vi "Dresden Edit Recipe(in).vi"() -> ()   [LabVIEW 2009] (continued)
                n2220 = local write "R Cmb Ch3 Target material"("Zn" ("R DC Target material")) -> ()
              }
              frame #97 {
                n2221 = local write "R Cmb Ch3 Target material"("ZnO" ("R DC Target material")) -> ()
              }
              frame #98 {
                n2222 = local write "R Cmb Ch3 Target material"("ZnSe" ("R DC Target material")) -> ()
              }
              frame #99 {
                n2223 = local write "R Cmb Ch3 Target material"("ZnS" ("R DC Target material")) -> ()
              }
              frame #100 {
                n2224 = local write "R Cmb Ch3 Target material"("Zr" ("R DC Target material")) -> ()
              }
              frame #101 {
                n2225 = local write "R Cmb Ch3 Target material"("ZrO2" ("R DC Target material")) -> ()
              }
              frame #102 {
                n2226 = local write "R Cmb Ch3 Target material"("Si3N4" ("R DC Target material")) -> ()
              }
              frame #103 {
                n2227 = local write "R Cmb Ch3 Target material"("ITO" ("R DC Target material")) -> ()
              }
              frame #104 {
                n2228 = local write "R Cmb Ch3 Target material"("PbI2" ("R DC Target material")) -> ()
              }
            }
            n2229 = local read "R Cmb Step9 Coating Power Active"() -> (w824:bool)
            n2230 = local read "R Cmb Step8 Coating Power Active"() -> (w825:bool)
            n2231 = case shown="True" w827 {
              frame #0 {
                w1044 = FALSE ("R Cmb Step3 Coating Power Active")
                n2232 = local write "R Cmb Step7 Coating Power Active"(w1044) -> ()
                n2233 = local write "R Cmb Step8 Coating Power Active"(w1044) -> ()
                n2234 = local write "R Cmb Step9 Coating Power Active"(w1044) -> ()
                n2235 = local write "R Cmb Step10 Coating Power Active"(w1044) -> ()
              }
              frame #1 {
                n2236 = local read "R Cmb Step7 Coating Power Active"() -> (w1045:bool)
                n2237 = case shown="False" w1045 {
                  frame #0 {
                    w1046 = 0.0 ("R Cmb Ch2 Step7 Coating Power")
                    w1047 = T5."Disabled and Grayed Out" ("Disabled")
                    n2238 = local write "R Cmb Ch3 Step7 Coating Power"(w1046) -> ()
                    n2239 = local write "R Cmb Ch2 Step7 Coating Power"(w1046) -> ()
                    n2240 = local write "R Cmb Interval length 7"(w1046) -> ()
                    n2241 = property on="R Cmb Ch3 Step7 Coating Power" class="DigNum (strict)"("DisabledEnum"=w1047) -> ()  [unwired: 2 in, 2 out]
                    n2242 = property on="R Cmb Interval length 7" class="DigNum (strict)"("DisabledEnum"=w1047) -> ()  [unwired: 2 in, 2 out]
                    n2243 = property on="R Cmb Ch2 Step7 Coating Power" class="DigNum (strict)"("DisabledEnum"=w1047) -> ()  [unwired: 2 in, 2 out]
                  }
                  frame #1 {
                    w1048 = T5."Enabled" ("Disabled")
                    n2244 = property on="R Cmb Ch3 Step7 Coating Power" class="DigNum (strict)"("DisabledEnum"=w1048) -> ()  [unwired: 2 in, 2 out]
                    n2245 = property on="R Cmb Interval length 7" class="DigNum (strict)"("DisabledEnum"=w1048) -> ()  [unwired: 2 in, 2 out]
                    n2246 = property on="R Cmb Ch2 Step7 Coating Power" class="DigNum (strict)"("DisabledEnum"=w1048) -> ()  [unwired: 2 in, 2 out]
                  }
                }
              }
            }
            n2247 = case shown="True" w826 {
              frame #0 {
                w1039 = FALSE ("R Cmb Step3 Coating Power Active")
                n2248 = local write "R Cmb Step8 Coating Power Active"(w1039) -> ()
                n2249 = local write "R Cmb Step9 Coating Power Active"(w1039) -> ()
                n2250 = local write "R Cmb Step10 Coating Power Active"(w1039) -> ()
              }
              frame #1 {
                n2251 = local read "R Cmb Step8 Coating Power Active"() -> (w1040:bool)
                n2252 = case shown="False" w1040 {
                  frame #0 {
                    w1041 = 0.0 ("R Cmb Ch2 Step8 Coating Power")
                    w1042 = T5."Disabled and Grayed Out" ("Disabled")
                    n2253 = local write "R Cmb Ch3 Step8 Coating Power"(w1041) -> ()
                    n2254 = local write "R Cmb Ch2 Step8 Coating Power"(w1041) -> ()
                    n2255 = local write "R Cmb Interval length 8"(w1041) -> ()
                    n2256 = property on="R Cmb Ch2 Step8 Coating Power" class="DigNum (strict)"("DisabledEnum"=w1042) -> ()  [unwired: 2 in, 2 out]
                    n2257 = property on="R Cmb Ch3 Step8 Coating Power" class="DigNum (strict)"("DisabledEnum"=w1042) -> ()  [unwired: 2 in, 2 out]
                    n2258 = property on="R Cmb Interval length 8" class="DigNum (strict)"("DisabledEnum"=w1042) -> ()  [unwired: 2 in, 2 out]
                  }
                  frame #1 {
                    w1043 = T5."Enabled" ("Disabled")
                    n2259 = property on="R Cmb Ch2 Step8 Coating Power" class="DigNum (strict)"("DisabledEnum"=w1043) -> ()  [unwired: 2 in, 2 out]
                    n2260 = property on="R Cmb Ch3 Step8 Coating Power" class="DigNum (strict)"("DisabledEnum"=w1043) -> ()  [unwired: 2 in, 2 out]
                    n2261 = property on="R Cmb Interval length 8" class="DigNum (strict)"("DisabledEnum"=w1043) -> ()  [unwired: 2 in, 2 out]
                  }
                }
              }
            }
            n2262 = case shown="True" w828 {
              frame #0 {
                w1049 = FALSE ("R Cmb Step3 Coating Power Active")
                n2263 = local write "R Cmb Step6 Coating Power Active"(w1049) -> ()
                n2264 = local write "R Cmb Step7 Coating Power Active"(w1049) -> ()
                n2265 = local write "R Cmb Step8 Coating Power Active"(w1049) -> ()
                n2266 = local write "R Cmb Step9 Coating Power Active"(w1049) -> ()
                n2267 = local write "R Cmb Step10 Coating Power Active"(w1049) -> ()
              }
              frame #1 {
                n2268 = local read "R Cmb Step6 Coating Power Active"() -> (w1050:bool)
                n2269 = case shown="False" w1050 {
                  frame #0 {
                    w1051 = 0.0 ("R Cmb Ch2 Step6 Coating Power")
                    w1052 = T5."Disabled and Grayed Out" ("Disabled")
                    n2270 = local write "R Cmb Ch2 Step6 Coating Power"(w1051) -> ()
                    n2271 = local write "R Cmb Ch3 Step6 Coating Power"(w1051) -> ()
                    n2272 = local write "R Cmb Interval length 6"(w1051) -> ()
                    n2273 = property on="R Cmb Ch2 Step6 Coating Power" class="DigNum (strict)"("DisabledEnum"=w1052) -> ()  [unwired: 2 in, 2 out]
                    n2274 = property on="R Cmb Ch3 Step6 Coating Power" class="DigNum (strict)"("DisabledEnum"=w1052) -> ()  [unwired: 2 in, 2 out]
                    n2275 = property on="R Cmb Interval length 6" class="DigNum (strict)"("DisabledEnum"=w1052) -> ()  [unwired: 2 in, 2 out]
                  }
                  frame #1 {
                    w1053 = T5."Enabled" ("Disabled")
                    n2276 = property on="R Cmb Ch2 Step6 Coating Power" class="DigNum (strict)"("DisabledEnum"=w1053) -> ()  [unwired: 2 in, 2 out]
                    n2277 = property on="R Cmb Ch3 Step6 Coating Power" class="DigNum (strict)"("DisabledEnum"=w1053) -> ()  [unwired: 2 in, 2 out]
                    n2278 = property on="R Cmb Interval length 6" class="DigNum (strict)"("DisabledEnum"=w1053) -> ()  [unwired: 2 in, 2 out]
                  }
                }
              }
            }
            n2279 = case shown="True" w824 {
              frame #0 {
                n2280 = local write "R Cmb Step10 Coating Power Active"(FALSE ("R Cmb Step3 Coating Power Active")) -> ()
              }
              frame #1 {
                n2281 = local read "R Cmb Step10 Coating Power Active"() -> (w1035:bool)
                n2282 = case shown="False" w1035 {
                  frame #0 {
                    w1036 = 0.0 ("R Cmb Ch2 Step10 Coating Power")
                    w1037 = T5."Disabled and Grayed Out" ("Disabled")
                    n2283 = local write "R Cmb Ch2 Step10 Coating Power"(w1036) -> ()
                    n2284 = local write "R Cmb Ch3 Step10 Coating Power"(w1036) -> ()
                    n2285 = local write "R Cmb Interval length 10"(w1036) -> ()
                    n2286 = property on="R Cmb Ch2 Step10 Coating Power" class="DigNum (strict)"("DisabledEnum"=w1037) -> ()  [unwired: 2 in, 2 out]
                    n2287 = property on="R Cmb Ch3 Step10 Coating Power" class="DigNum (strict)"("DisabledEnum"=w1037) -> ()  [unwired: 2 in, 2 out]
                    n2288 = property on="R Cmb Interval length 10" class="DigNum (strict)"("DisabledEnum"=w1037) -> ()  [unwired: 2 in, 2 out]
                  }
                  frame #1 {
                    w1038 = T5."Enabled" ("Disabled")
                    n2289 = property on="R Cmb Ch2 Step10 Coating Power" class="DigNum (strict)"("DisabledEnum"=w1038) -> ()  [unwired: 2 in, 2 out]
                    n2290 = property on="R Cmb Ch3 Step10 Coating Power" class="DigNum (strict)"("DisabledEnum"=w1038) -> ()  [unwired: 2 in, 2 out]
                    n2291 = property on="R Cmb Interval length 10" class="DigNum (strict)"("DisabledEnum"=w1038) -> ()  [unwired: 2 in, 2 out]
                  }
                }
              }
            }
            n2292 = case shown="True" w825 {
              frame #0 {
                w1029 = FALSE ("R Cmb Step3 Coating Power Active")
                n2293 = local write "R Cmb Step9 Coating Power Active"(w1029) -> ()
                n2294 = local write "R Cmb Step10 Coating Power Active"(w1029) -> ()
              }
              frame #1 {
                n2295 = local read "R Cmb Step9 Coating Power Active"() -> (w1030:bool)
                n2296 = case shown="False" w1030 {
                  frame #0 {
                    w1031 = 0.0 ("R Cmb Ch2 Step9 Coating Power")
                    w1032 = T5."Disabled and Grayed Out" ("Disabled")
                    n2297 = local write "R Cmb Ch3 Step9 Coating Power"(w1031) -> ()
                    n2298 = local write "R Cmb Ch2 Step9 Coating Power"(w1031) -> ()
                    n2299 = local write "R Cmb Interval length 9"(w1031) -> ()
                    n2300 = property on="R Cmb Ch2 Step9 Coating Power" class="DigNum (strict)"("DisabledEnum"=w1032) -> ()  [unwired: 2 in, 2 out]
                    n2301 = property on="R Cmb Ch3 Step9 Coating Power" class="DigNum (strict)"("DisabledEnum"=w1032) -> ()  [unwired: 2 in, 2 out]
                    n2302 = property on="R Cmb Interval length 9" class="DigNum (strict)"("DisabledEnum"=w1032) -> ()  [unwired: 2 in, 2 out]
                  }
                  frame #1 {
                    w1033 = T5."Enabled" ("Disabled")
                    n2303 = property on="R Cmb Ch2 Step9 Coating Power" class="DigNum (strict)"("DisabledEnum"=w1033) -> ()  [unwired: 2 in, 2 out]
                    n2304 = property on="R Cmb Ch3 Step9 Coating Power" class="DigNum (strict)"("DisabledEnum"=w1033) -> ()  [unwired: 2 in, 2 out]
                    n2305 = property on="R Cmb Interval length 9" class="DigNum (strict)"("DisabledEnum"=w1033) -> ()  [unwired: 2 in, 2 out]
                  }
                }
              }
            }
            n2306 = Or(x=w853, y="Cancel") -> (x .or. y?=w851:bool)
          }
        }
        frame #1 {
        }
      }
    }
  }
  "OKTO" <- w1
  n2307 = invoke class="VI" method="Default Vals.Reinit All"() -> (error out=w4:errorcluster)  [unwired: 3 in, 2 out]
  n2308 = property on="Recipe Name" class="Str"(error in=w4, "Key Focus"=TRUE) -> ()  [unwired: 1 in, 2 out]
  n2309 = case shown="True" w1 {
    tunnel: [errorcluster {"status"=FALSE, "code"=0, "source"=""} ("error out") w2514] -> w2
    frame #0 {
    }
    frame #1 {
      n2310 = stacked-sequence {
        seq-local: [w2521 _] -> [_ w2718]
        seq-local: [w2520 _] -> [_ w2714]
        seq-local: [w2519 _] -> [_ w2720]
        seq-local: [w2518 _] -> [_ w2715]
        seq-local: [w2516 _] -> [_ w2708]
        seq-local: [w2515 _] -> [_ w2711]
        tunnel: [_ w2719] -> w2514
        tunnel: [_ w2713] -> _
        tunnel: [_ w2710] -> _
        frame #0 {
          n2311 = File Dialog(9:"Recipe Name", 11:path "D:/System Files/Recipe" ("start path")) -> (3:w2528:path)  [unwired: 2 in, 6 out]
          n2312 = Build Path(base path=path "D:/System Files/Recipe" ("start path"), name or relative path="Recipe Name") -> (appended path=w2527:path)
          n2313 = Open/Create/Replace File(file path (use dialog)=w2527, operation (0:open)=T6."replace or create", access (0:read/write)=enum16{"read/write", "read-only", "write-only"}."read/write") -> (refnum out=w2518:refnum<file>, cancelled=w2525:bool, error out=w2523:errorcluster)  [unwired: 3 in]
          n2314 = Open/Create/Replace File(file path (use dialog)=w2528, operation (0:open)=T6."replace or create", access (0:read/write)=enum16{"read/write", "read-only", "write-only"}."read/write") -> (refnum out=w2519:refnum<file>, cancelled=w2531:bool, error out=w2533:errorcluster)  [unwired: 3 in]
          n2315 = stacked-sequence {
            tunnel: "Recipe Name" -> [_ w2539 _]
            tunnel: [_ w2538 _] -> w2516
            tunnel: [_ w2537 _] -> w2515
            frame #0 {
              n2316 = Wait (ms)(milliseconds to wait=u32 50) -> ()  [unwired: 1 out]
              n2317 = dll-call lib="kernel32.dll" fn="SetFileAttributesA"("lpFileName"="D:\\System Files\\Recipe Archive", "dwFileAttributes"=u32 128) -> ()  [unwired: 6 in, 2 out]
            }
            frame #1 {
              n2318 = Build Path(base path=path "D:/System Files/Recipe Archive" ("start path"), name or relative path=w2539) -> (appended path=w2540:path)
              n2319 = Open/Create/Replace File(file path (use dialog)=w2540, operation (0:open)=T6."replace or create", access (0:read/write)=enum16{"read/write", "read-only", "write-only"}."read/write") -> (refnum out=w2538:refnum<file>, cancelled=w2542:bool, error out=w2544:errorcluster)  [unwired: 3 in]
              n2320 = case shown="True" w2542 {
                tunnel: w2538 -> [_ w2549]
                tunnel: w2544 -> [_ w2548]
                tunnel: [errorcluster {"status"=FALSE, "code"=0, "source"=""} ("error out") w2547] -> w2537
                frame #0 {
                }
                frame #1 {
                  n2321 = Close File(refnum=w2549, error in=w2548) -> (error out=w2547:errorcluster)  [unwired: 1 out]
                }
              }
            }
            frame #2 {
              n2322 = Wait (ms)(milliseconds to wait=u32 50) -> ()  [unwired: 1 out]
              n2323 = dll-call lib="kernel32.dll" fn="SetFileAttributesA"("lpFileName"="D:\\System Files\\Recipe Archive", "dwFileAttributes"=u32 2) -> ()  [unwired: 6 in, 2 out]
            }
          }
          n2324 = case shown="False" w2525 {
            tunnel: w2518 -> [_ w2556]
            tunnel: w2523 -> [_ w2555]
            tunnel: [errorcluster {"status"=FALSE, "code"=0, "source"=""} ("error out") w2554] -> w2520
            frame #0 {
            }
            frame #1 {
              n2325 = Close File(refnum=w2556, error in=w2555) -> (error out=w2554:errorcluster)  [unwired: 1 out]
            }
          }
          n2326 = case shown="True" w2531 {
            tunnel: w2519 -> [_ w2560]
            tunnel: w2533 -> [_ w2559]
            tunnel: [errorcluster {"status"=FALSE, "code"=0, "source"=""} ("error out") w2558] -> w2521
            frame #0 {
            }
            frame #1 {
              n2327 = Close File(refnum=w2560, error in=w2559) -> (error out=w2558:errorcluster)  [unwired: 1 out]
            }
          }
        }
        frame #1 {
          n2328 = stacked-sequence {
            tunnel: [w2723 _ _ _ _ _ _ _ _ _ _ _ _ _ _ _ _ _ _ _ _ _ _ _ _ _ _ _ _ _ _ _ _ _ _ _ _ _ _ _ _ _ _ _ _ _ _ _ _ _ _ _ _ _ _ _ _ _ _ _ _ _ _ _ _ _ _ _ _ _ _ _ _ _ _ _ _ _ _ _ _ _ _ _ _ _ _ _ _ _ _ _ _ _ _ _ _ _ _ _ _ _ _ _ _ _ _ _ _ _ _ _ _ _ _ _ _ _ _ _ _ _ _ _ _ _ _ _ _ _ _ _ _ _ _ _ _ _ _ _ _ _ _ _ _ _] -> w2706
            tunnel: [_ w2730 _ _ _ _ _ _ _ _ _ _ _ _ _ _ _ _ _ _ _ _ _ _ _ _ _ _ _ _ _ _ _ _ _ _ _ _ _ _ _ _ _ _ _ _ _ _ _ _ _ _ _ _ _ _ _ _ _ _ _ _ _ _ _ _ _ _ _ _ _ _ _ _ _ _ _ _ _ _ _ _ _ _ _ _ _ _ _ _ _ _ _ _ _ _ _ _ _ _ _ _ _ _ _ _ _ _ _ _ _ _ _ _ _ _ _ _ _ _ _ _ _ _ _ _ _ _ _ _ _ _ _ _ _ _ _ _ _ _ _ _ _ _ _ _] -> w2705
            tunnel: [_ _ w2737 _ _ _ _ _ _ _ _ _ _ _ _ _ _ _ _ _ _ _ _ _ _ _ _ _ _ _ _ _ _ _ _ _ _ _ _ _ _ _ _ _ _ _ _ _ _ _ _ _ _ _ _ _ _ _ _ _ _ _ _ _ _ _ _ _ _ _ _ _ _ _ _ _ _ _ _ _ _ _ _ _ _ _ _ _ _ _ _ _ _ _ _ _ _ _ _ _ _ _ _ _ _ _ _ _ _ _ _ _ _ _ _ _ _ _ _ _ _ _ _ _ _ _ _ _ _ _ _ _ _ _ _ _ _ _ _ _ _ _ _ _ _ _] -> w2704
            tunnel: [_ _ _ w2746 _ _ _ _ _ _ _ _ _ _ _ _ _ _ _ _ _ _ _ _ _ _ _ _ _ _ _ _ _ _ _ _ _ _ _ _ _ _ _ _ _ _ _ _ _ _ _ _ _ _ _ _ _ _ _ _ _ _ _ _ _ _ _ _ _ _ _ _ _ _ _ _ _ _ _ _ _ _ _ _ _ _ _ _ _ _ _ _ _ _ _ _ _ _ _ _ _ _ _ _ _ _ _ _ _ _ _ _ _ _ _ _ _ _ _ _ _ _ _ _ _ _ _ _ _ _ _ _ _ _ _ _ _ _ _ _ _ _ _ _ _ _] -> w2703
            tunnel: [_ _ _ _ w2755 _ _ _ _ _ _ _ _ _ _ _ _ _ _ _ _ _ _ _ _ _ _ _ _ _ _ _ _ _ _ _ _ _ _ _ _ _ _ _ _ _ _ _ _ _ _ _ _ _ _ _ _ _ _ _ _ _ _ _ _ _ _ _ _ _ _ _ _ _ _ _ _ _ _ _ _ _ _ _ _ _ _ _ _ _ _ _ _ _ _ _ _ _ _ _ _ _ _ _ _ _ _ _ _ _ _ _ _ _ _ _ _ _ _ _ _ _ _ _ _ _ _ _ _ _ _ _ _ _ _ _ _ _ _ _ _ _ _ _ _ _] -> w2702
            tunnel: [_ _ _ _ _ w2759 _ _ _ _ _ _ _ _ _ _ _ _ _ _ _ _ _ _ _ _ _ _ _ _ _ _ _ _ _ _ _ _ _ _ _ _ _ _ _ _ _ _ _ _ _ _ _ _ _ _ _ _ _ _ _ _ _ _ _ _ _ _ _ _ _ _ _ _ _ _ _ _ _ _ _ _ _ _ _ _ _ _ _ _ _ _ _ _ _ _ _ _ _ _ _ _ _ _ _ _ _ _ _ _ _ _ _ _ _ _ _ _ _ _ _ _ _ _ _ _ _ _ _ _ _ _ _ _ _ _ _ _ _ _ _ _ _ _ _ _] -> w2701
            tunnel: [_ _ _ _ _ _ w2765 _ _ _ _ _ _ _ _ _ _ _ _ _ _ _ _ _ _ _ _ _ _ _ _ _ _ _ _ _ _ _ _ _ _ _ _ _ _ _ _ _ _ _ _ _ _ _ _ _ _ _ _ _ _ _ _ _ _ _ _ _ _ _ _ _ _ _ _ _ _ _ _ _ _ _ _ _ _ _ _ _ _ _ _ _ _ _ _ _ _ _ _ _ _ _ _ _ _ _ _ _ _ _ _ _ _ _ _ _ _ _ _ _ _ _ _ _ _ _ _ _ _ _ _ _ _ _ _ _ _ _ _ _ _ _ _ _ _ _] -> w2700
            tunnel: [_ _ _ _ _ _ _ w2771 _ _ _ _ _ _ _ _ _ _ _ _ _ _ _ _ _ _ _ _ _ _ _ _ _ _ _ _ _ _ _ _ _ _ _ _ _ _ _ _ _ _ _ _ _ _ _ _ _ _ _ _ _ _ _ _ _ _ _ _ _ _ _ _ _ _ _ _ _ _ _ _ _ _ _ _ _ _ _ _ _ _ _ _ _ _ _ _ _ _ _ _ _ _ _ _ _ _ _ _ _ _ _ _ _ _ _ _ _ _ _ _ _ _ _ _ _ _ _ _ _ _ _ _ _ _ _ _ _ _ _ _ _ _ _ _ _ _] -> w2699
            tunnel: [_ _ _ _ _ _ _ _ w2777 _ _ _ _ _ _ _ _ _ _ _ _ _ _ _ _ _ _ _ _ _ _ _ _ _ _ _ _ _ _ _ _ _ _ _ _ _ _ _ _ _ _ _ _ _ _ _ _ _ _ _ _ _ _ _ _ _ _ _ _ _ _ _ _ _ _ _ _ _ _ _ _ _ _ _ _ _ _ _ _ _ _ _ _ _ _ _ _ _ _ _ _ _ _ _ _ _ _ _ _ _ _ _ _ _ _ _ _ _ _ _ _ _ _ _ _ _ _ _ _ _ _ _ _ _ _ _ _ _ _ _ _ _ _ _ _ _] -> w2698
            tunnel: [_ _ _ _ _ _ _ _ _ w2783 _ _ _ _ _ _ _ _ _ _ _ _ _ _ _ _ _ _ _ _ _ _ _ _ _ _ _ _ _ _ _ _ _ _ _ _ _ _ _ _ _ _ _ _ _ _ _ _ _ _ _ _ _ _ _ _ _ _ _ _ _ _ _ _ _ _ _ _ _ _ _ _ _ _ _ _ _ _ _ _ _ _ _ _ _ _ _ _ _ _ _ _ _ _ _ _ _ _ _ _ _ _ _ _ _ _ _ _ _ _ _ _ _ _ _ _ _ _ _ _ _ _ _ _ _ _ _ _ _ _ _ _ _ _ _ _] -> w2697
            tunnel: [_ _ _ _ _ _ _ _ _ _ w2789 _ _ _ _ _ _ _ _ _ _ _ _ _ _ _ _ _ _ _ _ _ _ _ _ _ _ _ _ _ _ _ _ _ _ _ _ _ _ _ _ _ _ _ _ _ _ _ _ _ _ _ _ _ _ _ _ _ _ _ _ _ _ _ _ _ _ _ _ _ _ _ _ _ _ _ _ _ _ _ _ _ _ _ _ _ _ _ _ _ _ _ _ _ _ _ _ _ _ _ _ _ _ _ _ _ _ _ _ _ _ _ _ _ _ _ _ _ _ _ _ _ _ _ _ _ _ _ _ _ _ _ _ _ _ _] -> w2696
            tunnel: [_ _ _ _ _ _ _ _ _ _ _ w2796 _ _ _ _ _ _ _ _ _ _ _ _ _ _ _ _ _ _ _ _ _ _ _ _ _ _ _ _ _ _ _ _ _ _ _ _ _ _ _ _ _ _ _ _ _ _ _ _ _ _ _ _ _ _ _ _ _ _ _ _ _ _ _ _ _ _ _ _ _ _ _ _ _ _ _ _ _ _ _ _ _ _ _ _ _ _ _ _ _ _ _ _ _ _ _ _ _ _ _ _ _ _ _ _ _ _ _ _ _ _ _ _ _ _ _ _ _ _ _ _ _ _ _ _ _ _ _ _ _ _ _ _ _ _] -> w2695
            tunnel: [_ _ _ _ _ _ _ _ _ _ _ _ w2801 _ _ _ _ _ _ _ _ _ _ _ _ _ _ _ _ _ _ _ _ _ _ _ _ _ _ _ _ _ _ _ _ _ _ _ _ _ _ _ _ _ _ _ _ _ _ _ _ _ _ _ _ _ _ _ _ _ _ _ _ _ _ _ _ _ _ _ _ _ _ _ _ _ _ _ _ _ _ _ _ _ _ _ _ _ _ _ _ _ _ _ _ _ _ _ _ _ _ _ _ _ _ _ _ _ _ _ _ _ _ _ _ _ _ _ _ _ _ _ _ _ _ _ _ _ _ _ _ _ _ _ _ _] -> w2694
            tunnel: [_ _ _ _ _ _ _ _ _ _ _ _ _ w2809 _ _ _ _ _ _ _ _ _ _ _ _ _ _ _ _ _ _ _ _ _ _ _ _ _ _ _ _ _ _ _ _ _ _ _ _ _ _ _ _ _ _ _ _ _ _ _ _ _ _ _ _ _ _ _ _ _ _ _ _ _ _ _ _ _ _ _ _ _ _ _ _ _ _ _ _ _ _ _ _ _ _ _ _ _ _ _ _ _ _ _ _ _ _ _ _ _ _ _ _ _ _ _ _ _ _ _ _ _ _ _ _ _ _ _ _ _ _ _ _ _ _ _ _ _ _ _ _ _ _ _ _] -> w2693
            tunnel: [_ _ _ _ _ _ _ _ _ _ _ _ _ _ w2815 _ _ _ _ _ _ _ _ _ _ _ _ _ _ _ _ _ _ _ _ _ _ _ _ _ _ _ _ _ _ _ _ _ _ _ _ _ _ _ _ _ _ _ _ _ _ _ _ _ _ _ _ _ _ _ _ _ _ _ _ _ _ _ _ _ _ _ _ _ _ _ _ _ _ _ _ _ _ _ _ _ _ _ _ _ _ _ _ _ _ _ _ _ _ _ _ _ _ _ _ _ _ _ _ _ _ _ _ _ _ _ _ _ _ _ _ _ _ _ _ _ _ _ _ _ _ _ _ _ _ _] -> w2692
            tunnel: [_ _ _ _ _ _ _ _ _ _ _ _ _ _ _ w2822 _ _ _ _ _ _ _ _ _ _ _ _ _ _ _ _ _ _ _ _ _ _ _ _ _ _ _ _ _ _ _ _ _ _ _ _ _ _ _ _ _ _ _ _ _ _ _ _ _ _ _ _ _ _ _ _ _ _ _ _ _ _ _ _ _ _ _ _ _ _ _ _ _ _ _ _ _ _ _ _ _ _ _ _ _ _ _ _ _ _ _ _ _ _ _ _ _ _ _ _ _ _ _ _ _ _ _ _ _ _ _ _ _ _ _ _ _ _ _ _ _ _ _ _ _ _ _ _ _ _] -> w2691
            tunnel: [_ _ _ _ _ _ _ _ _ _ _ _ _ _ _ _ w2829 _ _ _ _ _ _ _ _ _ _ _ _ _ _ _ _ _ _ _ _ _ _ _ _ _ _ _ _ _ _ _ _ _ _ _ _ _ _ _ _ _ _ _ _ _ _ _ _ _ _ _ _ _ _ _ _ _ _ _ _ _ _ _ _ _ _ _ _ _ _ _ _ _ _ _ _ _ _ _ _ _ _ _ _ _ _ _ _ _ _ _ _ _ _ _ _ _ _ _ _ _ _ _ _ _ _ _ _ _ _ _ _ _ _ _ _ _ _ _ _ _ _ _ _ _ _ _ _ _] -> w2690
            tunnel: [_ _ _ _ _ _ _ _ _ _ _ _ _ _ _ _ _ w2837 _ _ _ _ _ _ _ _ _ _ _ _ _ _ _ _ _ _ _ _ _ _ _ _ _ _ _ _ _ _ _ _ _ _ _ _ _ _ _ _ _ _ _ _ _ _ _ _ _ _ _ _ _ _ _ _ _ _ _ _ _ _ _ _ _ _ _ _ _ _ _ _ _ _ _ _ _ _ _ _ _ _ _ _ _ _ _ _ _ _ _ _ _ _ _ _ _ _ _ _ _ _ _ _ _ _ _ _ _ _ _ _ _ _ _ _ _ _ _ _ _ _ _ _ _ _ _ _] -> w2689
            tunnel: [_ _ _ _ _ _ _ _ _ _ _ _ _ _ _ _ _ _ w2841 _ _ _ _ _ _ _ _ _ _ _ _ _ _ _ _ _ _ _ _ _ _ _ _ _ _ _ _ _ _ _ _ _ _ _ _ _ _ _ _ _ _ _ _ _ _ _ _ _ _ _ _ _ _ _ _ _ _ _ _ _ _ _ _ _ _ _ _ _ _ _ _ _ _ _ _ _ _ _ _ _ _ _ _ _ _ _ _ _ _ _ _ _ _ _ _ _ _ _ _ _ _ _ _ _ _ _ _ _ _ _ _ _ _ _ _ _ _ _ _ _ _ _ _ _ _ _] -> w2688
            tunnel: [_ _ _ _ _ _ _ _ _ _ _ _ _ _ _ _ _ _ _ w2847 _ _ _ _ _ _ _ _ _ _ _ _ _ _ _ _ _ _ _ _ _ _ _ _ _ _ _ _ _ _ _ _ _ _ _ _ _ _ _ _ _ _ _ _ _ _ _ _ _ _ _ _ _ _ _ _ _ _ _ _ _ _ _ _ _ _ _ _ _ _ _ _ _ _ _ _ _ _ _ _ _ _ _ _ _ _ _ _ _ _ _ _ _ _ _ _ _ _ _ _ _ _ _ _ _ _ _ _ _ _ _ _ _ _ _ _ _ _ _ _ _ _ _ _ _ _] -> w2687
            tunnel: [_ _ _ _ _ _ _ _ _ _ _ _ _ _ _ _ _ _ _ _ w2855 _ _ _ _ _ _ _ _ _ _ _ _ _ _ _ _ _ _ _ _ _ _ _ _ _ _ _ _ _ _ _ _ _ _ _ _ _ _ _ _ _ _ _ _ _ _ _ _ _ _ _ _ _ _ _ _ _ _ _ _ _ _ _ _ _ _ _ _ _ _ _ _ _ _ _ _ _ _ _ _ _ _ _ _ _ _ _ _ _ _ _ _ _ _ _ _ _ _ _ _ _ _ _ _ _ _ _ _ _ _ _ _ _ _ _ _ _ _ _ _ _ _ _ _ _] -> w2686
            tunnel: [_ _ _ _ _ _ _ _ _ _ _ _ _ _ _ _ _ _ _ _ _ w2860 _ _ _ _ _ _ _ _ _ _ _ _ _ _ _ _ _ _ _ _ _ _ _ _ _ _ _ _ _ _ _ _ _ _ _ _ _ _ _ _ _ _ _ _ _ _ _ _ _ _ _ _ _ _ _ _ _ _ _ _ _ _ _ _ _ _ _ _ _ _ _ _ _ _ _ _ _ _ _ _ _ _ _ _ _ _ _ _ _ _ _ _ _ _ _ _ _ _ _ _ _ _ _ _ _ _ _ _ _ _ _ _ _ _ _ _ _ _ _ _ _ _ _ _] -> w2685
            tunnel: [_ _ _ _ _ _ _ _ _ _ _ _ _ _ _ _ _ _ _ _ _ _ w2865 _ _ _ _ _ _ _ _ _ _ _ _ _ _ _ _ _ _ _ _ _ _ _ _ _ _ _ _ _ _ _ _ _ _ _ _ _ _ _ _ _ _ _ _ _ _ _ _ _ _ _ _ _ _ _ _ _ _ _ _ _ _ _ _ _ _ _ _ _ _ _ _ _ _ _ _ _ _ _ _ _ _ _ _ _ _ _ _ _ _ _ _ _ _ _ _ _ _ _ _ _ _ _ _ _ _ _ _ _ _ _ _ _ _ _ _ _ _ _ _ _ _ _] -> w2684
            tunnel: [_ _ _ _ _ _ _ _ _ _ _ _ _ _ _ _ _ _ _ _ _ _ _ w2875 _ _ _ _ _ _ _ _ _ _ _ _ _ _ _ _ _ _ _ _ _ _ _ _ _ _ _ _ _ _ _ _ _ _ _ _ _ _ _ _ _ _ _ _ _ _ _ _ _ _ _ _ _ _ _ _ _ _ _ _ _ _ _ _ _ _ _ _ _ _ _ _ _ _ _ _ _ _ _ _ _ _ _ _ _ _ _ _ _ _ _ _ _ _ _ _ _ _ _ _ _ _ _ _ _ _ _ _ _ _ _ _ _ _ _ _ _ _ _ _ _ _] -> w2683
            tunnel: [_ _ _ _ _ _ _ _ _ _ _ _ _ _ _ _ _ _ _ _ _ _ _ _ w2880 _ _ _ _ _ _ _ _ _ _ _ _ _ _ _ _ _ _ _ _ _ _ _ _ _ _ _ _ _ _ _ _ _ _ _ _ _ _ _ _ _ _ _ _ _ _ _ _ _ _ _ _ _ _ _ _ _ _ _ _ _ _ _ _ _ _ _ _ _ _ _ _ _ _ _ _ _ _ _ _ _ _ _ _ _ _ _ _ _ _ _ _ _ _ _ _ _ _ _ _ _ _ _ _ _ _ _ _ _ _ _ _ _ _ _ _ _ _ _ _ _] -> w2682
            tunnel: [_ _ _ _ _ _ _ _ _ _ _ _ _ _ _ _ _ _ _ _ _ _ _ _ _ w2889 _ _ _ _ _ _ _ _ _ _ _ _ _ _ _ _ _ _ _ _ _ _ _ _ _ _ _ _ _ _ _ _ _ _ _ _ _ _ _ _ _ _ _ _ _ _ _ _ _ _ _ _ _ _ _ _ _ _ _ _ _ _ _ _ _ _ _ _ _ _ _ _ _ _ _ _ _ _ _ _ _ _ _ _ _ _ _ _ _ _ _ _ _ _ _ _ _ _ _ _ _ _ _ _ _ _ _ _ _ _ _ _ _ _ _ _ _ _ _ _] -> w2681
            tunnel: [_ _ _ _ _ _ _ _ _ _ _ _ _ _ _ _ _ _ _ _ _ _ _ _ _ _ w2895 _ _ _ _ _ _ _ _ _ _ _ _ _ _ _ _ _ _ _ _ _ _ _ _ _ _ _ _ _ _ _ _ _ _ _ _ _ _ _ _ _ _ _ _ _ _ _ _ _ _ _ _ _ _ _ _ _ _ _ _ _ _ _ _ _ _ _ _ _ _ _ _ _ _ _ _ _ _ _ _ _ _ _ _ _ _ _ _ _ _ _ _ _ _ _ _ _ _ _ _ _ _ _ _ _ _ _ _ _ _ _ _ _ _ _ _ _ _ _] -> w2680
            tunnel: [_ _ _ _ _ _ _ _ _ _ _ _ _ _ _ _ _ _ _ _ _ _ _ _ _ _ _ w2901 _ _ _ _ _ _ _ _ _ _ _ _ _ _ _ _ _ _ _ _ _ _ _ _ _ _ _ _ _ _ _ _ _ _ _ _ _ _ _ _ _ _ _ _ _ _ _ _ _ _ _ _ _ _ _ _ _ _ _ _ _ _ _ _ _ _ _ _ _ _ _ _ _ _ _ _ _ _ _ _ _ _ _ _ _ _ _ _ _ _ _ _ _ _ _ _ _ _ _ _ _ _ _ _ _ _ _ _ _ _ _ _ _ _ _ _ _ _] -> w2679
            tunnel: [_ _ _ _ _ _ _ _ _ _ _ _ _ _ _ _ _ _ _ _ _ _ _ _ _ _ _ _ w2910 _ _ _ _ _ _ _ _ _ _ _ _ _ _ _ _ _ _ _ _ _ _ _ _ _ _ _ _ _ _ _ _ _ _ _ _ _ _ _ _ _ _ _ _ _ _ _ _ _ _ _ _ _ _ _ _ _ _ _ _ _ _ _ _ _ _ _ _ _ _ _ _ _ _ _ _ _ _ _ _ _ _ _ _ _ _ _ _ _ _ _ _ _ _ _ _ _ _ _ _ _ _ _ _ _ _ _ _ _ _ _ _ _ _ _ _ _] -> w2678
            tunnel: [_ _ _ _ _ _ _ _ _ _ _ _ _ _ _ _ _ _ _ _ _ _ _ _ _ _ _ _ _ w2916 _ _ _ _ _ _ _ _ _ _ _ _ _ _ _ _ _ _ _ _ _ _ _ _ _ _ _ _ _ _ _ _ _ _ _ _ _ _ _ _ _ _ _ _ _ _ _ _ _ _ _ _ _ _ _ _ _ _ _ _ _ _ _ _ _ _ _ _ _ _ _ _ _ _ _ _ _ _ _ _ _ _ _ _ _ _ _ _ _ _ _ _ _ _ _ _ _ _ _ _ _ _ _ _ _ _ _ _ _ _ _ _ _ _ _ _] -> w2677
            tunnel: [_ _ _ _ _ _ _ _ _ _ _ _ _ _ _ _ _ _ _ _ _ _ _ _ _ _ _ _ _ _ w2922 _ _ _ _ _ _ _ _ _ _ _ _ _ _ _ _ _ _ _ _ _ _ _ _ _ _ _ _ _ _ _ _ _ _ _ _ _ _ _ _ _ _ _ _ _ _ _ _ _ _ _ _ _ _ _ _ _ _ _ _ _ _ _ _ _ _ _ _ _ _ _ _ _ _ _ _ _ _ _ _ _ _ _ _ _ _ _ _ _ _ _ _ _ _ _ _ _ _ _ _ _ _ _ _ _ _ _ _ _ _ _ _ _ _ _] -> w2676
            tunnel: [_ _ _ _ _ _ _ _ _ _ _ _ _ _ _ _ _ _ _ _ _ _ _ _ _ _ _ _ _ _ _ w2932 _ _ _ _ _ _ _ _ _ _ _ _ _ _ _ _ _ _ _ _ _ _ _ _ _ _ _ _ _ _ _ _ _ _ _ _ _ _ _ _ _ _ _ _ _ _ _ _ _ _ _ _ _ _ _ _ _ _ _ _ _ _ _ _ _ _ _ _ _ _ _ _ _ _ _ _ _ _ _ _ _ _ _ _ _ _ _ _ _ _ _ _ _ _ _ _ _ _ _ _ _ _ _ _ _ _ _ _ _ _ _ _ _ _] -> w2675
            tunnel: [_ _ _ _ _ _ _ _ _ _ _ _ _ _ _ _ _ _ _ _ _ _ _ _ _ _ _ _ _ _ _ _ w2937 _ _ _ _ _ _ _ _ _ _ _ _ _ _ _ _ _ _ _ _ _ _ _ _ _ _ _ _ _ _ _ _ _ _ _ _ _ _ _ _ _ _ _ _ _ _ _ _ _ _ _ _ _ _ _ _ _ _ _ _ _ _ _ _ _ _ _ _ _ _ _ _ _ _ _ _ _ _ _ _ _ _ _ _ _ _ _ _ _ _ _ _ _ _ _ _ _ _ _ _ _ _ _ _ _ _ _ _ _ _ _ _ _] -> w2674
            tunnel: [_ _ _ _ _ _ _ _ _ _ _ _ _ _ _ _ _ _ _ _ _ _ _ _ _ _ _ _ _ _ _ _ _ w2943 _ _ _ _ _ _ _ _ _ _ _ _ _ _ _ _ _ _ _ _ _ _ _ _ _ _ _ _ _ _ _ _ _ _ _ _ _ _ _ _ _ _ _ _ _ _ _ _ _ _ _ _ _ _ _ _ _ _ _ _ _ _ _ _ _ _ _ _ _ _ _ _ _ _ _ _ _ _ _ _ _ _ _ _ _ _ _ _ _ _ _ _ _ _ _ _ _ _ _ _ _ _ _ _ _ _ _ _ _ _ _ _] -> w2673
            tunnel: [_ _ _ _ _ _ _ _ _ _ _ _ _ _ _ _ _ _ _ _ _ _ _ _ _ _ _ _ _ _ _ _ _ _ w2953 _ _ _ _ _ _ _ _ _ _ _ _ _ _ _ _ _ _ _ _ _ _ _ _ _ _ _ _ _ _ _ _ _ _ _ _ _ _ _ _ _ _ _ _ _ _ _ _ _ _ _ _ _ _ _ _ _ _ _ _ _ _ _ _ _ _ _ _ _ _ _ _ _ _ _ _ _ _ _ _ _ _ _ _ _ _ _ _ _ _ _ _ _ _ _ _ _ _ _ _ _ _ _ _ _ _ _ _ _ _ _] -> w2672
            tunnel: [_ _ _ _ _ _ _ _ _ _ _ _ _ _ _ _ _ _ _ _ _ _ _ _ _ _ _ _ _ _ _ _ _ _ _ w2958 _ _ _ _ _ _ _ _ _ _ _ _ _ _ _ _ _ _ _ _ _ _ _ _ _ _ _ _ _ _ _ _ _ _ _ _ _ _ _ _ _ _ _ _ _ _ _ _ _ _ _ _ _ _ _ _ _ _ _ _ _ _ _ _ _ _ _ _ _ _ _ _ _ _ _ _ _ _ _ _ _ _ _ _ _ _ _ _ _ _ _ _ _ _ _ _ _ _ _ _ _ _ _ _ _ _ _ _ _ _] -> w2671
            tunnel: [_ _ _ _ _ _ _ _ _ _ _ _ _ _ _ _ _ _ _ _ _ _ _ _ _ _ _ _ _ _ _ _ _ _ _ _ w2964 _ _ _ _ _ _ _ _ _ _ _ _ _ _ _ _ _ _ _ _ _ _ _ _ _ _ _ _ _ _ _ _ _ _ _ _ _ _ _ _ _ _ _ _ _ _ _ _ _ _ _ _ _ _ _ _ _ _ _ _ _ _ _ _ _ _ _ _ _ _ _ _ _ _ _ _ _ _ _ _ _ _ _ _ _ _ _ _ _ _ _ _ _ _ _ _ _ _ _ _ _ _ _ _ _ _ _ _ _] -> w2670
            tunnel: [_ _ _ _ _ _ _ _ _ _ _ _ _ _ _ _ _ _ _ _ _ _ _ _ _ _ _ _ _ _ _ _ _ _ _ _ _ w2974 _ _ _ _ _ _ _ _ _ _ _ _ _ _ _ _ _ _ _ _ _ _ _ _ _ _ _ _ _ _ _ _ _ _ _ _ _ _ _ _ _ _ _ _ _ _ _ _ _ _ _ _ _ _ _ _ _ _ _ _ _ _ _ _ _ _ _ _ _ _ _ _ _ _ _ _ _ _ _ _ _ _ _ _ _ _ _ _ _ _ _ _ _ _ _ _ _ _ _ _ _ _ _ _ _ _ _ _] -> w2669
            tunnel: [_ _ _ _ _ _ _ _ _ _ _ _ _ _ _ _ _ _ _ _ _ _ _ _ _ _ _ _ _ _ _ _ _ _ _ _ _ _ w2979 _ _ _ _ _ _ _ _ _ _ _ _ _ _ _ _ _ _ _ _ _ _ _ _ _ _ _ _ _ _ _ _ _ _ _ _ _ _ _ _ _ _ _ _ _ _ _ _ _ _ _ _ _ _ _ _ _ _ _ _ _ _ _ _ _ _ _ _ _ _ _ _ _ _ _ _ _ _ _ _ _ _ _ _ _ _ _ _ _ _ _ _ _ _ _ _ _ _ _ _ _ _ _ _ _ _ _] -> w2668
            tunnel: [_ _ _ _ _ _ _ _ _ _ _ _ _ _ _ _ _ _ _ _ _ _ _ _ _ _ _ _ _ _ _ _ _ _ _ _ _ _ _ w2985 _ _ _ _ _ _ _ _ _ _ _ _ _ _ _ _ _ _ _ _ _ _ _ _ _ _ _ _ _ _ _ _ _ _ _ _ _ _ _ _ _ _ _ _ _ _ _ _ _ _ _ _ _ _ _ _ _ _ _ _ _ _ _ _ _ _ _ _ _ _ _ _ _ _ _ _ _ _ _ _ _ _ _ _ _ _ _ _ _ _ _ _ _ _ _ _ _ _ _ _ _ _ _ _ _ _] -> w2667
            tunnel: [_ _ _ _ _ _ _ _ _ _ _ _ _ _ _ _ _ _ _ _ _ _ _ _ _ _ _ _ _ _ _ _ _ _ _ _ _ _ _ _ w2995 _ _ _ _ _ _ _ _ _ _ _ _ _ _ _ _ _ _ _ _ _ _ _ _ _ _ _ _ _ _ _ _ _ _ _ _ _ _ _ _ _ _ _ _ _ _ _ _ _ _ _ _ _ _ _ _ _ _ _ _ _ _ _ _ _ _ _ _ _ _ _ _ _ _ _ _ _ _ _ _ _ _ _ _ _ _ _ _ _ _ _ _ _ _ _ _ _ _ _ _ _ _ _ _ _] -> w2666
            tunnel: [_ _ _ _ _ _ _ _ _ _ _ _ _ _ _ _ _ _ _ _ _ _ _ _ _ _ _ _ _ _ _ _ _ _ _ _ _ _ _ _ _ w3000 _ _ _ _ _ _ _ _ _ _ _ _ _ _ _ _ _ _ _ _ _ _ _ _ _ _ _ _ _ _ _ _ _ _ _ _ _ _ _ _ _ _ _ _ _ _ _ _ _ _ _ _ _ _ _ _ _ _ _ _ _ _ _ _ _ _ _ _ _ _ _ _ _ _ _ _ _ _ _ _ _ _ _ _ _ _ _ _ _ _ _ _ _ _ _ _ _ _ _ _ _ _ _ _] -> w2665
            tunnel: [_ _ _ _ _ _ _ _ _ _ _ _ _ _ _ _ _ _ _ _ _ _ _ _ _ _ _ _ _ _ _ _ _ _ _ _ _ _ _ _ _ _ w3006 _ _ _ _ _ _ _ _ _ _ _ _ _ _ _ _ _ _ _ _ _ _ _ _ _ _ _ _ _ _ _ _ _ _ _ _ _ _ _ _ _ _ _ _ _ _ _ _ _ _ _ _ _ _ _ _ _ _ _ _ _ _ _ _ _ _ _ _ _ _ _ _ _ _ _ _ _ _ _ _ _ _ _ _ _ _ _ _ _ _ _ _ _ _ _ _ _ _ _ _ _ _ _] -> w2664
            tunnel: [_ _ _ _ _ _ _ _ _ _ _ _ _ _ _ _ _ _ _ _ _ _ _ _ _ _ _ _ _ _ _ _ _ _ _ _ _ _ _ _ _ _ _ w3016 _ _ _ _ _ _ _ _ _ _ _ _ _ _ _ _ _ _ _ _ _ _ _ _ _ _ _ _ _ _ _ _ _ _ _ _ _ _ _ _ _ _ _ _ _ _ _ _ _ _ _ _ _ _ _ _ _ _ _ _ _ _ _ _ _ _ _ _ _ _ _ _ _ _ _ _ _ _ _ _ _ _ _ _ _ _ _ _ _ _ _ _ _ _ _ _ _ _ _ _ _ _] -> w2663
            tunnel: [_ _ _ _ _ _ _ _ _ _ _ _ _ _ _ _ _ _ _ _ _ _ _ _ _ _ _ _ _ _ _ _ _ _ _ _ _ _ _ _ _ _ _ _ w3021 _ _ _ _ _ _ _ _ _ _ _ _ _ _ _ _ _ _ _ _ _ _ _ _ _ _ _ _ _ _ _ _ _ _ _ _ _ _ _ _ _ _ _ _ _ _ _ _ _ _ _ _ _ _ _ _ _ _ _ _ _ _ _ _ _ _ _ _ _ _ _ _ _ _ _ _ _ _ _ _ _ _ _ _ _ _ _ _ _ _ _ _ _ _ _ _ _ _ _ _ _] -> w2662
            tunnel: [_ _ _ _ _ _ _ _ _ _ _ _ _ _ _ _ _ _ _ _ _ _ _ _ _ _ _ _ _ _ _ _ _ _ _ _ _ _ _ _ _ _ _ _ _ w3027 _ _ _ _ _ _ _ _ _ _ _ _ _ _ _ _ _ _ _ _ _ _ _ _ _ _ _ _ _ _ _ _ _ _ _ _ _ _ _ _ _ _ _ _ _ _ _ _ _ _ _ _ _ _ _ _ _ _ _ _ _ _ _ _ _ _ _ _ _ _ _ _ _ _ _ _ _ _ _ _ _ _ _ _ _ _ _ _ _ _ _ _ _ _ _ _ _ _ _ _] -> w2661
            tunnel: [_ _ _ _ _ _ _ _ _ _ _ _ _ _ _ _ _ _ _ _ _ _ _ _ _ _ _ _ _ _ _ _ _ _ _ _ _ _ _ _ _ _ _ _ _ _ w3037 _ _ _ _ _ _ _ _ _ _ _ _ _ _ _ _ _ _ _ _ _ _ _ _ _ _ _ _ _ _ _ _ _ _ _ _ _ _ _ _ _ _ _ _ _ _ _ _ _ _ _ _ _ _ _ _ _ _ _ _ _ _ _ _ _ _ _ _ _ _ _ _ _ _ _ _ _ _ _ _ _ _ _ _ _ _ _ _ _ _ _ _ _ _ _ _ _ _ _] -> w2660
            tunnel: [_ _ _ _ _ _ _ _ _ _ _ _ _ _ _ _ _ _ _ _ _ _ _ _ _ _ _ _ _ _ _ _ _ _ _ _ _ _ _ _ _ _ _ _ _ _ _ w3042 _ _ _ _ _ _ _ _ _ _ _ _ _ _ _ _ _ _ _ _ _ _ _ _ _ _ _ _ _ _ _ _ _ _ _ _ _ _ _ _ _ _ _ _ _ _ _ _ _ _ _ _ _ _ _ _ _ _ _ _ _ _ _ _ _ _ _ _ _ _ _ _ _ _ _ _ _ _ _ _ _ _ _ _ _ _ _ _ _ _ _ _ _ _ _ _ _ _] -> w2659
            tunnel: [_ _ _ _ _ _ _ _ _ _ _ _ _ _ _ _ _ _ _ _ _ _ _ _ _ _ _ _ _ _ _ _ _ _ _ _ _ _ _ _ _ _ _ _ _ _ _ _ w3048 _ _ _ _ _ _ _ _ _ _ _ _ _ _ _ _ _ _ _ _ _ _ _ _ _ _ _ _ _ _ _ _ _ _ _ _ _ _ _ _ _ _ _ _ _ _ _ _ _ _ _ _ _ _ _ _ _ _ _ _ _ _ _ _ _ _ _ _ _ _ _ _ _ _ _ _ _ _ _ _ _ _ _ _ _ _ _ _ _ _ _ _ _ _ _ _ _] -> w2658
            tunnel: [_ _ _ _ _ _ _ _ _ _ _ _ _ _ _ _ _ _ _ _ _ _ _ _ _ _ _ _ _ _ _ _ _ _ _ _ _ _ _ _ _ _ _ _ _ _ _ _ _ w3057 _ _ _ _ _ _ _ _ _ _ _ _ _ _ _ _ _ _ _ _ _ _ _ _ _ _ _ _ _ _ _ _ _ _ _ _ _ _ _ _ _ _ _ _ _ _ _ _ _ _ _ _ _ _ _ _ _ _ _ _ _ _ _ _ _ _ _ _ _ _ _ _ _ _ _ _ _ _ _ _ _ _ _ _ _ _ _ _ _ _ _ _ _ _ _ _] -> w2657
            tunnel: [_ _ _ _ _ _ _ _ _ _ _ _ _ _ _ _ _ _ _ _ _ _ _ _ _ _ _ _ _ _ _ _ _ _ _ _ _ _ _ _ _ _ _ _ _ _ _ _ _ _ w3063 _ _ _ _ _ _ _ _ _ _ _ _ _ _ _ _ _ _ _ _ _ _ _ _ _ _ _ _ _ _ _ _ _ _ _ _ _ _ _ _ _ _ _ _ _ _ _ _ _ _ _ _ _ _ _ _ _ _ _ _ _ _ _ _ _ _ _ _ _ _ _ _ _ _ _ _ _ _ _ _ _ _ _ _ _ _ _ _ _ _ _ _ _ _ _] -> w2656
            tunnel: [_ _ _ _ _ _ _ _ _ _ _ _ _ _ _ _ _ _ _ _ _ _ _ _ _ _ _ _ _ _ _ _ _ _ _ _ _ _ _ _ _ _ _ _ _ _ _ _ _ _ _ w3069 _ _ _ _ _ _ _ _ _ _ _ _ _ _ _ _ _ _ _ _ _ _ _ _ _ _ _ _ _ _ _ _ _ _ _ _ _ _ _ _ _ _ _ _ _ _ _ _ _ _ _ _ _ _ _ _ _ _ _ _ _ _ _ _ _ _ _ _ _ _ _ _ _ _ _ _ _ _ _ _ _ _ _ _ _ _ _ _ _ _ _ _ _ _] -> w2655
            tunnel: [_ _ _ _ _ _ _ _ _ _ _ _ _ _ _ _ _ _ _ _ _ _ _ _ _ _ _ _ _ _ _ _ _ _ _ _ _ _ _ _ _ _ _ _ _ _ _ _ _ _ _ _ w3079 _ _ _ _ _ _ _ _ _ _ _ _ _ _ _ _ _ _ _ _ _ _ _ _ _ _ _ _ _ _ _ _ _ _ _ _ _ _ _ _ _ _ _ _ _ _ _ _ _ _ _ _ _ _ _ _ _ _ _ _ _ _ _ _ _ _ _ _ _ _ _ _ _ _ _ _ _ _ _ _ _ _ _ _ _ _ _ _ _ _ _ _ _] -> w2654
